vi "Interpolate Oversampled Data.vi"(10 "Bits of Precision Increase":i32, 11 "Waveform in":waveform(dbl)) -> (3 "Waveform out":waveform(dbl))   [LabVIEW 2021]
doc: "Applies an interpolation algorithm to the data, to smoothe and filter the results.\n\nIncreasing the bit rate (resolution of magnitude measurements) reduces the sample rate (measurements / second)"
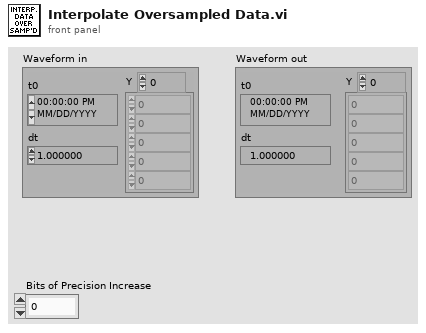
[diagram p1: front panel]
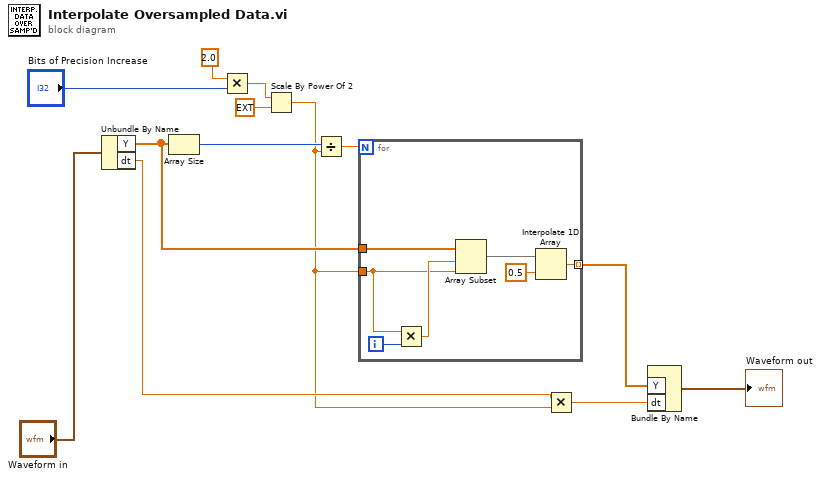
[diagram p0: block diagram]
diagram:
  n1 = Unbundle By Name("Waveform in") -> ("Y"=w9:dbl[], "dt"=w11:dbl)
  n2 = Array Size(array=w9) -> (size(s)=w6:i32)
  n3 = Multiply(x=2.0, y="Bits of Precision Increase") -> (x*y=w5:dbl)
  n4 = Scale By Power Of 2(n=w5, x=ext 1.0) -> (x*2^n=w2:ext)
  n5 = Divide(x=w6, y=w2) -> (x/y=w7:ext)
  n6 = for {
    N: w7 -> [_]
    tunnel: w9 -> [w19]
    tunnel: [w15] -> w10 mode=indexing
    tunnel: w2 -> [w14]
    i -> [w20]
    n7 = Multiply(x=w14, y=w20) -> (x*y=w18:ext)
    n8 = Array Subset(array=w19, index=w18, length=w14) -> (w17:dbl[])
    n9 = Interpolate 1D Array(1:0.5 ("fractional index or x"), 2:w17) -> (0:w15:dbl)
  }
  n10 = Multiply(x=w11, y=w2) -> (x*y=w12:ext)
  n11 = Bundle By Name("Y"=w10, "dt"=w12) -> (→"Waveform out":waveform(dbl))  [unwired: 1 in]
